vi "setShooterSpeed.vi"(0 "CAN Talon SRX Ref":T1={"DeviceStatus"={"status"=FALSE, "code"=0, "source"=""}, "Type"=enum."PWM", "PWM"={"PWM Channel"=enum."PWM 1", "DeadBand"={"Name"="", "maxPositivePwm"=0, "minPositivePwm"=0, "centerPwm"=0, "maxNegativePwm"=0, "minNegativePwm"=0, "angularRange"=0}}, "CAN"={"Device Number"=0, "Control Mode"=enum."Percent VBus", "Semaphore"=refnum, "Max Vout"=12.0, "TalonSRX Control Mode"=enum."Percent VBus"}, "Invert"=FALSE}, 1 "Encoder Codes Per Rev":u16=256, 5 "array":bool[](array[boolean]), 7 "Intake Button":i32=4, 9 "Shoot Button":i32=4, 11 "Reverse Button":i32=4) -> ()   [LabVIEW 2015]
uses:
  <vilib>/Rock Robotics/WPI/MotorControl/WPI_MotorControlDeviceRef.ctl
  <vilib>/Rock Robotics/WPI/MotorControl/WPI_MotorControlType.ctl
  <vilib>/Rock Robotics/SystemInterfaces/DIO/FPGA_DIOPWMChannel.ctl
  <vilib>/Rock Robotics/WPI/PWM/WPI_PWMDeadband.ctl
  <vilib>/Rock Robotics/WPI/CAN/Jaguar/SubVIs/WPI_CANJaguar_ControlMode.ctl
  <vilib>/Rock Robotics/WPI/CAN/TalonSRX/WPI_CANTalonSRX_APIControlMode.ctl
  <vilib>/Rock Robotics/WPI/CAN/TalonSRX/WPI_CANTalonSRX_APIFeedbackSelect.ctl
panel:
  in  "Intake Speed":dbl(slide)=5349.794238683128 scale=0.0..10000.0
  in  "top speed":dbl(slide)=19520.0 scale=0.0..20000.0
  in  "F":dbl=0.12359
  in  "P":dbl(slide)=0.14345549738219895 scale=0.0..0.2
  out "Error":dbl
  out "Sensor Velocity":dbl
  out "Encoder B Pin State":bool
  out "Encoder A Pin State":bool
  out "Encoder Velocity":dbl
  out "Feedback Chart":cluster{dbl, dbl}(graph)={-0.0, 0.0}
  out "Actual Speed (RPM)":dbl(knob)=-0.0 scale=-2500.0..20000.0 scale format="%4d"
  in  "Set Speed (RPM)":dbl(slide) scale=-2500.0..10000.0
  in  "Reverse Feedback Sensor":bool=TRUE
  # ".143, 0, 0, .1235"
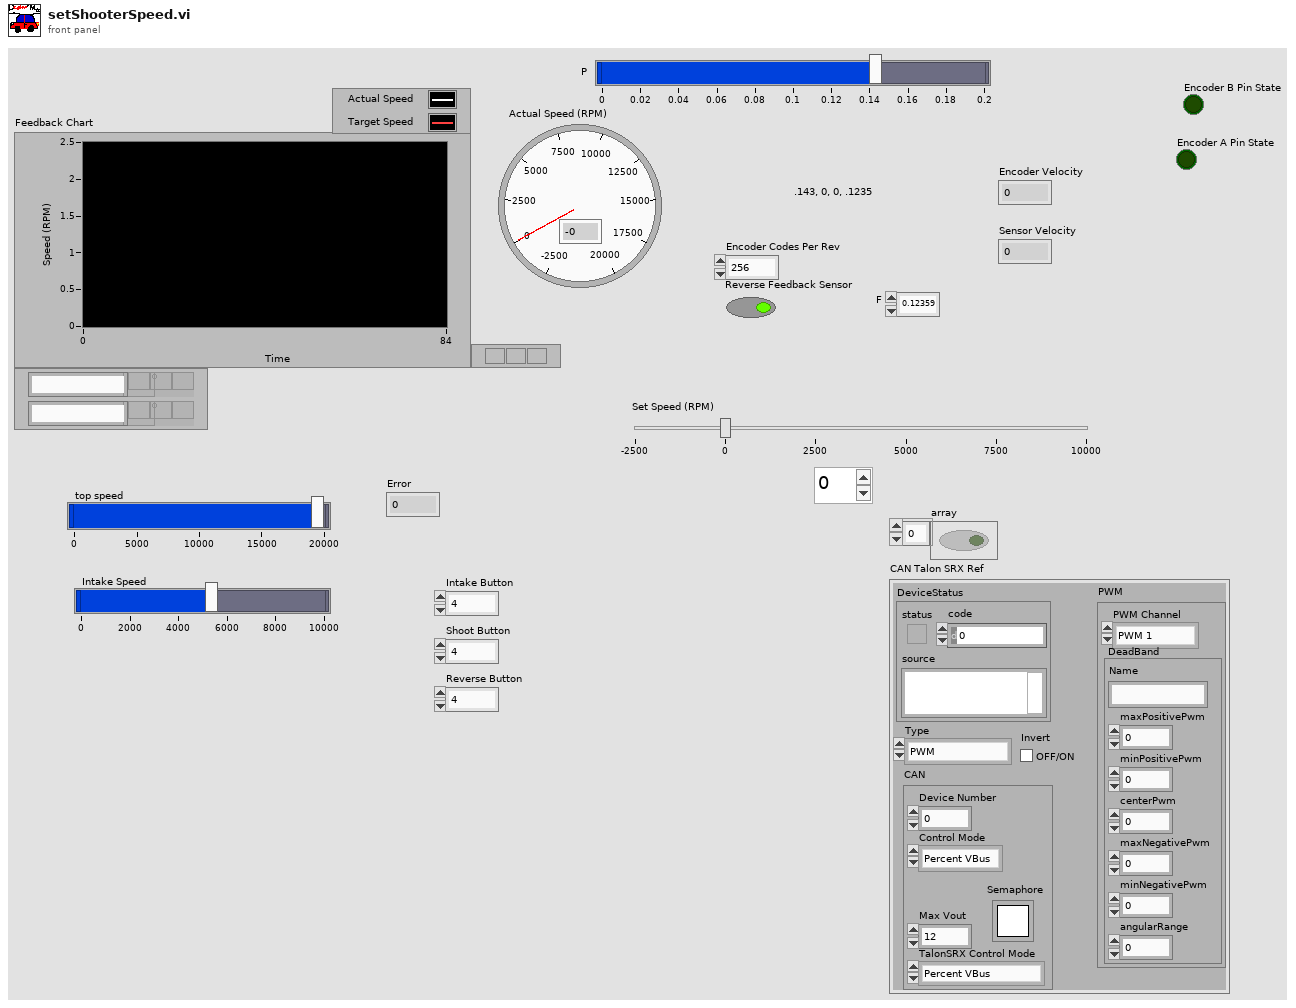
[diagram p1: front panel]
types:
  T1 = typedef "WPI_MotorControlDeviceRef.ctl" = cluster{"DeviceStatus":errorcluster, "Type":T2, "PWM":cluster{"PWM Channel":T3, "DeadBand":T4}, "CAN":cluster{"Device Number":u8, "Control Mode":T5, "Semaphore":T6, "Max Vout":dbl, "TalonSRX Control Mode":T7}, "Invert":bool}
  T2 = typedef "WPI_MotorControlType.ctl" = enum16{"PWM", "CAN", "CANTalonSRX"}
  T3 = typedef "FPGA_DIOPWMChannel.ctl" = enum8{"PWM 0", "PWM 1", "PWM 2", "PWM 3", "PWM 4", "PWM 5", "PWM 6", "PWM 7", "PWM 8", "PWM 9", "PWM MXP 0", "PWM MXP 1", "PWM MXP 2", "PWM MXP 3", "PWM MXP 4", "PWM MXP 5", "PWM MXP 6", "PWM MXP 7", "PWM MXP 8", "PWM MXP 9", "Invalid"}
  T4 = typedef "WPI_PWMDeadband.ctl" = cluster{"Name":string, "maxPositivePwm":i32, "minPositivePwm":i32, "centerPwm":i32, "maxNegativePwm":i32, "minNegativePwm":i32, "angularRange":u16}
  T5 = typedef "WPI_CANJaguar_ControlMode.ctl" = enum8{"Percent VBus", "Current", "Speed", "Position", "Voltage"}
  T6 = typedef "Semaphore RefNum" = refnum<k1>
  T7 = typedef "WPI_CANTalonSRX_APIControlMode.ctl" = enum8{"Percent VBus", "Speed", "Position", "Slave", "Unchanged / Invalid", "Voltage Compensation", "Current", "Motion Profile"}
  T8 = typedef "WPI_CANTalonSRX_APIFeedbackSelect.ctl" = enum16{"Digital Quadrature Encoder", "Analog Potentiometer", "Analog Encoder", "Count on Quad-A (Rising-Edge)", "Count on Quad-A (Falling-Edge)", "CTR Magnetic Enc (Absolute)", "CTR Magnetic Enc (Relative)", "Pulse Width"}
  T9 = typedef "WPI_CANTalonSRX_GlobalStatus.ctl" = cluster{"Applied Throttle":dbl, "Module Enabled":bool, "CAN Error":errorcluster, "Closed Loop Error":dbl, "Forward Limit Switch Closed":bool, "Reverse Limit Switch Closed":bool, "Sensor Position":dbl, "Sensor Velocity":dbl, "Current":dbl, "Sticky Fault - Over Temp":bool, "Sticky Fault - Under Voltage":bool, "Sticky Fault - Forward Limit":bool, "Sticky Fault - Reverse Limit":bool, "Sticky Fault - Forward Soft Limit":bool, "Sticky Fault - Reverse Soft Limit":bool, "Brake is Enabled":bool, "Encoder Position":dbl, "Encoder Velocity":dbl, "Encoder Index Count":dbl, "Encoder A Pin State":bool, "Encoder B Pin State":bool, "Encoder Index Pin State":bool, "Analog In":dbl, "Analog In Velocity":dbl, "Temperature (C)":dbl, "Battery Voltage":dbl, "Control 5 Is Supported":bool, "Current Profile Slot Select":dbl, "Pos Div 8":bool, "Vel Div 4":bool, "Pulse Width Position":i32, "Pulse Width Velocity":i32, "Pulse Width Rise To Rise (us)":i32, "Pulse Width Rise To Fall (us)":i32, "Mot Prof Active Is Under Run":bool, "Mot Prof Active Has Under Run":bool, "Mot Prof Active Is Last":bool, "Mot Prof Active Velocity Only":bool, "Mot Prof Active Is Valid":bool, "Mot Prof Buffer Is Full":bool, "Mot Prof Active Profile Slot Select":i32, "Mot Prof NextID":i32, "Mot Prof Count":i32, "Mot Prof Active Velocity":dbl, "Mot Prof Active Position":dbl, "Mot Prof Output Enable":i32}
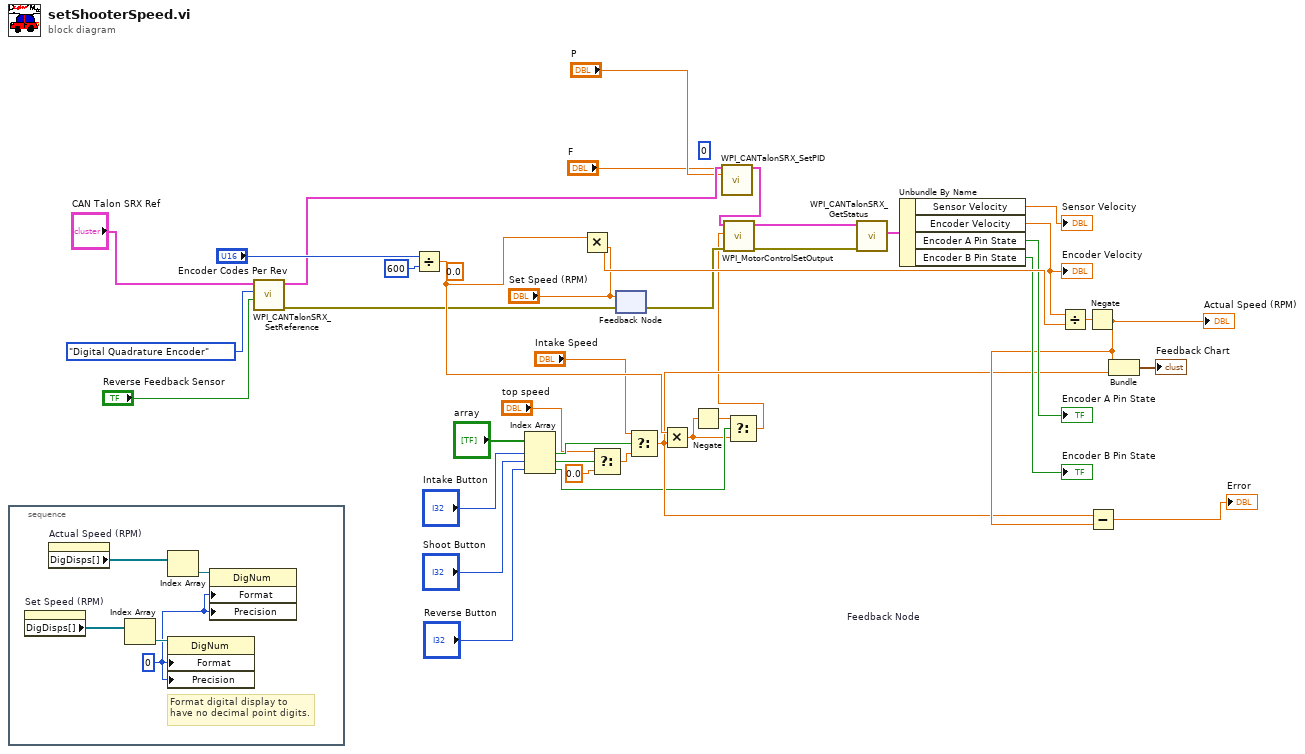
[diagram p0: block diagram]
diagram:
  (unwired) u8 0 ("Parameter Slot")
  (unwired) 0.0
  n1 = stacked-sequence {
    frame #0 {
      w39 = u8 0 ("Display Format:Format")
      # "Format digital display to have no decimal point digits."
      n2 = property on="Set Speed (RPM)" class="Slide (strict)"() -> ("DigDisps[]"=w40:refnum<vi>[])  [unwired: 2 in, 2 out]
      n3 = property on="Actual Speed (RPM)" class="Knob (strict)"() -> ("DigDisps[]"=w43:refnum<vi>[])  [unwired: 2 in, 2 out]
      n4 = Index Array(array=w40) -> (element=w41:refnum<vi>)  [unwired: 1 in]
      n5 = Index Array(array=w43) -> (element=w42:refnum<vi>)  [unwired: 1 in]
      n6 = property class="DigNum"(reference=w41, "Format"=w39, "Precision"=w39) -> ()  [unwired: 1 in, 2 out]
      n7 = property class="DigNum"(reference=w42, "Format"=w39, "Precision"=w39) -> ()  [unwired: 1 in, 2 out]
    }
  }
  n8 = call <vilib>:"WPI_CANTalonSRX_SetReference.vi"("Reverse Feedback Sensor"="Reverse Feedback Sensor", "Feedback Reference"=WPI_CANTalonSRX_APIFeedbackSelect."Digital Quadrature Encoder", "CAN Talon SRX Ref"="CAN Talon SRX Ref") -> ("error out"=w34:errorcluster, "CAN Talon SRX Ref"=w32:T1)  [unwired: 7 in]
  n9 = Divide(x="Encoder Codes Per Rev", y=u16 600) -> (x/y=w37:dbl)
  n10 = Index Array(array="array", index #1="Intake Button", index #2="Shoot Button", index #3="Reverse Button") -> (element #1=w22:bool, element #2=w20:bool, element #3=w8:bool)
  n11 = Multiply(x=w37, y="Set Speed (RPM)") -> ()  [unwired: 1 out]
  n12 = Select(t="top speed", s=w20, f=0.0) -> (s? t:f=w18:dbl)
  n13 = feedback #1 "Feedback Node"() -> ()  [unwired: 2 in]
  n14 = feedback-in #1("Set Speed (RPM)") -> ()
  n15 = Select(t="Intake Speed", s=w22, f=w18) -> (s? t:f=w10:dbl)
  n16 = Multiply(x=w37, y=w10) -> (x*y=w7:dbl)
  n17 = Negate(x=w7) -> (-x=w5:dbl)
  n18 = call <vilib>:"WPI_CANTalonSRX_SetPID.vi"("CAN Talon SRX Ref"=w32, "P"="P", "F"="F") -> ("CAN Talon SRX Ref"=w14:T1)  [unwired: 11 in, 1 out]
  n19 = Select(t=w5, s=w8, f=w7) -> (s? t:f=w6:dbl)
  n20 = call <vilib>:"WPI_MotorControlSetOutput.vi"("error in (no error)"=w34, "Output"=w6, "MotorControlDevRef"=w14) -> ("error out"=w26:errorcluster, "MotorControlDevRef"=w31:T1)  [unwired: 6 in, 1 out]
  n21 = call <vilib>:"WPI_CANTalonSRX_GetStatus.vi"("error in (no error)"=w26, "CAN Talon SRX Ref"=w31) -> ("Talon SRX Status"=w30:T9)  [unwired: 7 in, 2 out]
  n22 = Unbundle By Name(w30) -> ("Sensor Velocity"=→"Sensor Velocity":dbl, "Encoder Velocity"=w29:dbl, "Encoder A Pin State"=→"Encoder A Pin State":bool, "Encoder B Pin State"=→"Encoder B Pin State":bool)
  "Encoder Velocity" <- w29
  n23 = Divide(x=w29, y=w37) -> (x/y=w28:dbl)
  n24 = Negate(x=w28) -> (-x=w13:dbl)
  "Actual Speed (RPM)" <- w13
  n25 = Subtract(x=w10, y=w13) -> (x-y=→"Error":dbl)
  n26 = Bundle(w13, "f"=w10) -> (→"Feedback Chart":cluster{dbl, "f":dbl})  [unwired: 1 in]
